vi "诊断标定4.vi"(8 "CAN端口":u16(ring), 9 "设备索引号":u16(ring), 10 "CAN卡类型":u32(ring)=4) -> ()   [LabVIEW 2013] (continued)
                                n824 = Bundle By Name(cluster=w1320, "电池串联"=w1318, "电池并联"=w1318, "电池包额定容量"=w1318, "电池包额定能量"=w1318, "电池包额定总电压"=w1318, "实际容量"=w1318, "电池厂家"=w1317, "电池类型"=w1317, "电池生产日期"=w1317) -> (w1319:T12)
                                n825 = local write "电池信息"(w1319) -> ()
                                }
                                frame "电池包组号" {
                                n826 = local read "电池信息"() -> (w1323:T12)
                                n827 = Bundle By Name(cluster=w1323, "电池包组号"="") -> (w1322:T12)
                                n828 = local write "电池信息"(w1322) -> ()
                                }
                                frame "充放电安时" {
                                w1324 = 0.0 ("累计充电总安时")
                                n829 = local read "电池信息"() -> (w1326:T12)
                                n830 = Bundle By Name(cluster=w1326, "累计充电总安时"=w1324, "累计放电总安时"=w1324) -> (w1325:T12)
                                n831 = local write "电池信息"(w1325) -> ()
                                }
                                frame "电池充放电次数" {
                                w1327 = 0.0 ("累计充电总安时")
                                n832 = local read "电池信息"() -> (w1329:T12)
                                n833 = Bundle By Name(cluster=w1329, "电池充满次数"=w1327, "电池放空次数"=w1327, "电池充电次数"=w1327) -> (w1328:T12)
                                n834 = local write "电池信息"(w1328) -> ()
                                }
                              }
                            }
                            frame "从板" {
                              n835 = case shown="\"保险位置\"" w1330 {
                                frame "假", Default {
                                }
                                frame "电压起始值" {
                                n836 = control-ref of="项目信息 2"() -> (w1331:refnum<vi>)
                                n837 = for {
                                N: 2 -> [_]
                                tunnel: [""] -> w1335 mode=indexing
                                }
                                n838 = call "表格数据输入-8.6.vi"("行数"=u32 0, "列数"=u32 1, "字符串数组"=w1335, "表格引用"=w1331) -> ()  [unwired: 8 in]
                                }
                                frame "通道电压个数" {
                                n839 = control-ref of="项目信息 2"() -> (w1337:refnum<vi>)
                                n840 = for {
                                N: 20 -> [_]
                                tunnel: [""] -> w1341 mode=indexing
                                }
                                n841 = call "表格数据输入-8.6.vi"("行数"=u32 2, "列数"=u32 1, "字符串数组"=w1341, "表格引用"=w1337) -> ()  [unwired: 8 in]
                                }
                                frame "保险位置" {
                                n842 = control-ref of="项目信息 2"() -> (w1343:refnum<vi>)
                                n843 = for {
                                N: 10 -> [_]
                                tunnel: [""] -> w1347 mode=indexing
                                }
                                n844 = call "表格数据输入-8.6.vi"("行数"=u32 24, "列数"=u32 1, "字符串数组"=w1347, "表格引用"=w1343) -> ()  [unwired: 8 in]
                                }
                                frame "温度起始值" {
                                n845 = control-ref of="项目信息 2"() -> (w1349:refnum<vi>)
                                n846 = for {
                                N: 2 -> [_]
                                tunnel: [""] -> w1353 mode=indexing
                                }
                                n847 = call "表格数据输入-8.6.vi"("行数"=u32 22, "列数"=u32 1, "字符串数组"=w1353, "表格引用"=w1349) -> ()  [unwired: 8 in]
                                }
                                frame "加热控制参数" {
                                n848 = local write "加热控制参数"(T10 {"风机开启温度"=0.0, "风机关闭温度"=0.0, "加热开启温度"=0.0, "加热关闭温度"=0.0, "风机开启温差"=0.0, "风机关闭温差"=0.0, "加热关闭温差"=0.0} ("加热控制参数")) -> ()
                                }
                                frame "一级故障阀值" {
                                n849 = local write "一级故障 6"(T14 {"电压过高"=0.0, "电压过低"=0.0, "温度过高"=0.0, "温度过低"=0.0, "电压不均衡(V)"=0.0, "温度不均衡"=0.0, "SOC过低"=0.0} ("一级故障 6")) -> ()
                                }
                                frame "二级故障阀值" {
                                n850 = local write "一级故障 7"(T14 {"电压过高"=0.0, "电压过低"=0.0, "温度过高"=0.0, "温度过低"=0.0, "电压不均衡(V)"=0.0, "温度不均衡"=0.0, "SOC过低"=0.0} ("一级故障 7")) -> ()
                                }
                                frame "三级故障阀值" {
                                n851 = local write "一级故障 8"(T14 {"电压过高"=0.0, "电压过低"=0.0, "温度过高"=0.0, "温度过低"=0.0, "电压不均衡(V)"=0.0, "温度不均衡"=0.0, "SOC过低"=0.0} ("一级故障 7")) -> ()
                                }
                              }
                            }
                          }
                        }
                        frame #1 {
                          n852 = call <vilib>:"Set Busy.vi"("disable click? (T)"=FALSE) -> ()  [unwired: 3 in, 8 out]
                          n853 = global write "EV05全局变量1.vi" "写入超时"(FALSE ("写入超时")) -> ()
                          n854 = Wait Until Next ms Multiple(millisecond multiple=u32 50 ("毫秒倍数")) -> ()  [unwired: 1 out]
                          n855 = global write "EV05全局变量1.vi" "流控帧 2"(FALSE ("流控帧 2")) -> ()
                          n856 = local write "控制1"(TRUE ("控制1")) -> ()
                          n857 = local write "写?"(FALSE ("写?")) -> ()
                          n858 = local write "消除"(TRUE ("消除")) -> ()
                        }
                        frame #2 {
                          n859 = local read "设备索引号"() -> (w1367:u16)
                          n860 = local read "CAN卡类型"() -> (w1368:u32)
                          n861 = local write "命令序号"(w1371) -> ()
                          n862 = local read "CAN端口"() -> (w1366:u16)
                          n863 = stacked-sequence {
                            tunnel: w1372 -> [_ w1383]
                            tunnel: w1371 -> [_ w1382]
                            tunnel: w1370 -> [_ w1381]
                            tunnel: w1369 -> [_ w1380]
                            tunnel: w1368 -> [w1375 w1379]
                            tunnel: w1367 -> [w1374 w1378]
                            tunnel: w1366 -> [w1373 w1377]
                            frame #0 {
                              n864 = dll-call lib="PTH1Aabs EEV05EV05监控上位机-EV05EV05data\nusbcan.dll" fn="VCI_ClearBuffer"("DeviceType"=w1375, "DeviceInd"=w1374, "CANInd"=w1373) -> (error out=w1376:errorcluster)  [unwired: 4 in, 4 out]
                              n865 = call <vilib>:"Clear Errors.vi"("error in (no error)"=w1376) -> ()  [unwired: 6 in, 1 out]
                            }
                            frame #1 {
                              n866 = call "多帧发送机制(EV05).vi"("can卡类型"=w1379, "设备索引号"=w1378, "CAN端口"=w1377, "命令"=w1383, "板号"=w1381, "命令序号"=w1382, "输入数据"=w1380) -> ()  [unwired: 1 in, 12 out]
                            }
                          }
                        }
                        frame #3 {
                          n867 = while {
                            tunnel: [w1388] -> w1385
                            tunnel: [w1387] -> w1384
                            i -> [w1391]
                            stop <- w1388 stop-if-true
                            n868 = local read "强制停止"() -> (w1386:bool)
                            n869 = global read "EV05全局变量1.vi" "写入超时"() -> (w1387:bool)
                            n870 = Greater Or Equal?(x=w1391, y=25) -> (x >= y?=w1389:bool)
                            n871 = Compound Arithmetic op=OR(w1386, w1387, w1389) -> (w1388:bool)
                            n872 = Wait Until Next ms Multiple(millisecond multiple=u32 100 ("毫秒倍数")) -> ()  [unwired: 1 out]
                          }
                        }
                        frame #4 {
                          n873 = call <vilib>:"Unset Busy.vi"() -> ()  [unwired: 2 in, 10 out]
                          n874 = case shown="假" w1394 {
                            tunnel: w1393 -> [w1395 _]
                            frame False {
                              n875 = control-ref of="结果"() -> (w1397:refnum<vi>)
                              n876 = Concatenate Strings(w1395, "     读取失败" ("字符串")) -> (w1399:string)
                              n877 = Build Array(w1399) -> (w1396:string[])
                              n878 = call "表格编辑.vi"("新元素/子数组"=w1396, "活动单元格:单元格背景色"=u32 16740749, "MCListbox引用句柄"=w1397) -> ()  [unwired: 9 out]
                            }
                            frame True {
                            }
                          }
                        }
                        frame #5 {
                          n879 = And(x=w1401, y=w1403) -> (x .and. y?=w1402:bool)
                          n880 = case shown="真" w1402 {
                            frame False {
                            }
                            frame True {
                              n881 = local write "强制停止"(FALSE ("强制停止")) -> ()
                              n882 = control-ref of="结果"() -> (w1406:refnum<vi>)
                              n883 = Concatenate Strings("读取完成" ("字符串")) -> (w1408:string)
                              n884 = Build Array(w1408) -> (w1405:string[])
                              n885 = call "表格编辑.vi"("新元素/子数组"=w1405, "活动单元格:单元格背景色"=u32 21937, "MCListbox引用句柄"=w1406) -> ()  [unwired: 9 out]
                            }
                          }
                        }
                      }
                    }
                    n886 = local read "强制停止"() -> (w1217:bool)
                    n887 = Or(x=w1217, y=w1216) -> (x .or. y?=w1214:bool)
                  }
                }
              }
              frame #2 {
                n888 = case shown="假" w1488 {
                  tunnel: w1489 -> [w1490 _]
                  frame False {
                    n889 = case shown="\"从板\"" w1490 {
                      frame "主板", Default {
                        n890 = global read "读配置文件全局.vi" "电池额定实际容量判定"() -> (w1504:bool)
                        n891 = global read "读配置文件全局.vi" "电池充放电次数判定"() -> (w1493:bool)
                        n892 = global read "读配置文件全局.vi" "加热控制参数判定"() -> (w1491:bool)
                        n893 = global read "读配置文件全局.vi" "配置文件版本判定"() -> (w1503:bool)
                        n894 = global read "读配置文件全局.vi" "充电控制参数判定"() -> (w1497:bool)
                        n895 = global read "读配置文件全局.vi" "通道电压数判定"() -> (w1509:bool)
                        n896 = global read "读配置文件全局.vi" "电压起始值判定"() -> (w1508:bool)
                        n897 = global read "读配置文件全局.vi" "温度起始值判定"() -> (w1506:bool)
                        n898 = global read "读配置文件全局.vi" "充放电安时判定"() -> (w1495:bool)
                        n899 = global read "读配置文件全局.vi" "电池包组号判定"() -> (w1494:bool)
                        n900 = global read "读配置文件全局.vi" "电池信息1判定"() -> (w1496:bool)
                        n901 = global read "读配置文件全局.vi" "从板个数判定"() -> (w1512:bool)
                        n902 = global read "读配置文件全局.vi" "产品编号判定"() -> (w1511:bool)
                        n903 = global read "读配置文件全局.vi" "电压个数判定"() -> (w1510:bool)
                        n904 = global read "读配置文件全局.vi" "温度个数判定"() -> (w1507:bool)
                        n905 = global read "读配置文件全局.vi" "保险位置判定"() -> (w1505:bool)
                        n906 = global read "读配置文件全局.vi" "一级故障判定"() -> (w1500:bool)
                        n907 = global read "读配置文件全局.vi" "二级故障判定"() -> (w1499:bool)
                        n908 = global read "读配置文件全局.vi" "三级故障判定"() -> (w1498:bool)
                        n909 = global read "读配置文件全局.vi" "车牌号判定"() -> (w1502:bool)
                        n910 = global read "读配置文件全局.vi" "SOH判定"() -> (w1501:bool)
                        n911 = Build Array(w1512, w1511, w1510, w1509, w1508, w1507, w1506, w1505, w1504, w1503, w1502, w1501, w1500, w1499, w1498, w1497, w1496, w1495, w1494, w1493, w1491) -> (w1492:bool[])
                        n912 = And Array Elements(Boolean array=w1492) -> (logical AND=w1513:bool)
                        n913 = disable-structure shown="禁用" {
                          frame Disabled {
                            n914 = global read "读配置文件全局.vi" "SOC判定"() -> ()  [unwired: 1 out]
                          }
                          frame Enabled {
                          }
                        }
                        n915 = case shown="假" w1513 {
                          tunnel: w1492 -> [_ w1518]
                          frame True {
                            n916 = control-ref of="结果"() -> (w1516:refnum<vi>)
                            n917 = Build Array("全部判定成功!!!!!!!!") -> (w1517:string[])
                            n918 = call "表格编辑.vi"("新元素/子数组"=w1517, "活动单元格:单元格背景色"=u32 6618880, "MCListbox引用句柄"=w1516) -> ()  [unwired: 9 out]
                          }
                          frame False {
                            n919 = stacked-sequence {
                              tunnel: w1518 -> [_ w1523]
                              frame #0 {
                                n920 = control-ref of="结果"() -> (w1521:refnum<vi>)
                                n921 = Build Array("全部判定失败!!!!!") -> (w1522:string[])
                                n922 = call "表格编辑.vi"("新元素/子数组"=w1522, "活动单元格:单元格背景色"=u32 16711680, "MCListbox引用句柄"=w1521) -> ()  [unwired: 9 out]
                              }
                              frame #1 {
                                n923 = for {
                                tunnel: w1523 -> [w1525] mode=indexing
                                i -> [w1524]
                                n924 = case shown="20" w1524 {
                                tunnel: w1525 -> [w1526 w1531 w1536 w1541 w1546 w1551 w1556 w1561 w1566 w1571 w1576 w1581 w1586 w1591 w1596 w1601 w1606 w1611 w1616 w1621 w1626 _]
                                frame 0 {
                                n925 = case shown="假" w1526 {
                                frame False {
                                n926 = control-ref of="结果"() -> (w1529:refnum<vi>)
                                n927 = Build Array("从板个数判定失败!") -> (w1530:string[])
                                n928 = call "表格编辑.vi"("新元素/子数组"=w1530, "活动单元格:单元格背景色"=u32 16711680, "MCListbox引用句柄"=w1529) -> ()  [unwired: 9 out]
                                }
                                frame True {
                                }
                                }
                                }
                                frame 1 {
                                n929 = case shown="假" w1531 {
                                frame False {
                                n930 = control-ref of="结果"() -> (w1534:refnum<vi>)
                                n931 = Build Array("产品编号判定失败!") -> (w1535:string[])
                                n932 = call "表格编辑.vi"("新元素/子数组"=w1535, "活动单元格:单元格背景色"=u32 16711680, "MCListbox引用句柄"=w1534) -> ()  [unwired: 9 out]
                                }
                                frame True {
                                }
                                }
                                }
                                frame 2 {
                                n933 = case shown="假" w1536 {
                                frame False {
                                n934 = control-ref of="结果"() -> (w1539:refnum<vi>)
                                n935 = Build Array("电压个数判定失败!") -> (w1540:string[])
                                n936 = call "表格编辑.vi"("新元素/子数组"=w1540, "活动单元格:单元格背景色"=u32 16711680, "MCListbox引用句柄"=w1539) -> ()  [unwired: 9 out]
                                }
                                frame True {
                                }
                                }
                                }
                                frame 3 {
                                n937 = case shown="假" w1541 {
                                frame False {
                                n938 = control-ref of="结果"() -> (w1544:refnum<vi>)
                                n939 = Build Array("通道电压数判定失败!") -> (w1545:string[])
                                n940 = call "表格编辑.vi"("新元素/子数组"=w1545, "活动单元格:单元格背景色"=u32 16711680, "MCListbox引用句柄"=w1544) -> ()  [unwired: 9 out]
                                }
                                frame True {
                                }
                                }
                                }
                                frame 4 {
                                n941 = case shown="假" w1546 {
                                frame False {
                                n942 = control-ref of="结果"() -> (w1549:refnum<vi>)
                                n943 = Build Array("电压起始值判定失败!") -> (w1550:string[])
                                n944 = call "表格编辑.vi"("新元素/子数组"=w1550, "活动单元格:单元格背景色"=u32 16711680, "MCListbox引用句柄"=w1549) -> ()  [unwired: 9 out]
                                }
                                frame True {
                                }
                                }
                                }
                                frame 5 {
                                n945 = case shown="假" w1551 {
                                frame False {
                                n946 = control-ref of="结果"() -> (w1554:refnum<vi>)
                                n947 = Build Array("温度个数判定失败!") -> (w1555:string[])
                                n948 = call "表格编辑.vi"("新元素/子数组"=w1555, "活动单元格:单元格背景色"=u32 16711680, "MCListbox引用句柄"=w1554) -> ()  [unwired: 9 out]
                                }
                                frame True {
                                }
                                }
                                }
                                frame 6 {
                                n949 = case shown="假" w1556 {
                                frame False {
                                n950 = control-ref of="结果"() -> (w1559:refnum<vi>)
                                n951 = Build Array("温度起始值判定失败!") -> (w1560:string[])
                                n952 = call "表格编辑.vi"("新元素/子数组"=w1560, "活动单元格:单元格背景色"=u32 16711680, "MCListbox引用句柄"=w1559) -> ()  [unwired: 9 out]
                                }
                                frame True {
                                }
                                }
                                }
                                frame 7 {
                                n953 = case shown="假" w1561 {
                                frame False {
                                n954 = control-ref of="结果"() -> (w1564:refnum<vi>)
                                n955 = Build Array("保险位置判定失败!") -> (w1565:string[])
                                n956 = call "表格编辑.vi"("新元素/子数组"=w1565, "活动单元格:单元格背景色"=u32 16711680, "MCListbox引用句柄"=w1564) -> ()  [unwired: 9 out]
                                }
                                frame True {
                                }
                                }
                                }
                                frame 8 {
                                n957 = case shown="假" w1566 {
                                frame False {
                                n958 = control-ref of="结果"() -> (w1569:refnum<vi>)
                                n959 = Build Array("电池额定实际容量判定失败!") -> (w1570:string[])
                                n960 = call "表格编辑.vi"("新元素/子数组"=w1570, "活动单元格:单元格背景色"=u32 16711680, "MCListbox引用句柄"=w1569) -> ()  [unwired: 9 out]
                                }
                                frame True {
                                }
                                }
                                }
                                frame 9 {
                                n961 = case shown="假" w1571 {
                                frame False {
                                n962 = control-ref of="结果"() -> (w1574:refnum<vi>)
                                n963 = Build Array("配置文件版本判定失败!") -> (w1575:string[])
                                n964 = call "表格编辑.vi"("新元素/子数组"=w1575, "活动单元格:单元格背景色"=u32 16711680, "MCListbox引用句柄"=w1574) -> ()  [unwired: 9 out]
                                }
                                frame True {
                                }
                                }
                                }
                                frame 10 {
                                n965 = case shown="假" w1576 {
                                frame False {
                                n966 = control-ref of="结果"() -> (w1579:refnum<vi>)
                                n967 = Build Array("车牌号判定失败!") -> (w1580:string[])
                                n968 = call "表格编辑.vi"("新元素/子数组"=w1580, "活动单元格:单元格背景色"=u32 16711680, "MCListbox引用句柄"=w1579) -> ()  [unwired: 9 out]
                                }
                                frame True {
                                }
                                }
                                }
                                frame 11 {
                                n969 = case shown="假" w1581 {
                                frame False {
                                n970 = control-ref of="结果"() -> (w1584:refnum<vi>)
                                n971 = Build Array("SOH判定失败!") -> (w1585:string[])
                                n972 = call "表格编辑.vi"("新元素/子数组"=w1585, "活动单元格:单元格背景色"=u32 16711680, "MCListbox引用句柄"=w1584) -> ()  [unwired: 9 out]
                                }
                                frame True {
                                }
                                }
                                }
                                frame 12 {
                                n973 = case shown="假" w1586 {
                                frame False {
                                n974 = control-ref of="结果"() -> (w1589:refnum<vi>)
                                n975 = Build Array("一级故障阀值判定失败!") -> (w1590:string[])
                                n976 = call "表格编辑.vi"("新元素/子数组"=w1590, "活动单元格:单元格背景色"=u32 16711680, "MCListbox引用句柄"=w1589) -> ()  [unwired: 9 out]
                                }
                                frame True {
                                }
                                }
                                }
                                frame 13 {
                                n977 = case shown="假" w1591 {
                                frame False {
                                n978 = control-ref of="结果"() -> (w1594:refnum<vi>)
                                n979 = Build Array("二级故障阀值判定失败!") -> (w1595:string[])
                                n980 = call "表格编辑.vi"("新元素/子数组"=w1595, "活动单元格:单元格背景色"=u32 16711680, "MCListbox引用句柄"=w1594) -> ()  [unwired: 9 out]
                                }
                                frame True {
                                }
                                }
                                }
                                frame 14 {
                                n981 = case shown="假" w1596 {
                                frame False {
                                n982 = control-ref of="结果"() -> (w1599:refnum<vi>)
                                n983 = Build Array("三级故障阀值判定失败!") -> (w1600:string[])
                                n984 = call "表格编辑.vi"("新元素/子数组"=w1600, "活动单元格:单元格背景色"=u32 16711680, "MCListbox引用句柄"=w1599) -> ()  [unwired: 9 out]
                                }
                                frame True {
                                }
                                }
                                }
                                frame 15 {
                                n985 = case shown="假" w1601 {
                                frame False {
                                n986 = control-ref of="结果"() -> (w1604:refnum<vi>)
                                n987 = Build Array("充电控制参数判定失败!") -> (w1605:string[])
                                n988 = call "表格编辑.vi"("新元素/子数组"=w1605, "活动单元格:单元格背景色"=u32 16711680, "MCListbox引用句柄"=w1604) -> ()  [unwired: 9 out]
                                }
                                frame True {
                                }
                                }
                                }
                                frame 16 {
                                n989 = case shown="假" w1606 {
                                frame False {
                                n990 = control-ref of="结果"() -> (w1609:refnum<vi>)
                                n991 = Build Array("电池信息1判定失败!") -> (w1610:string[])
                                n992 = call "表格编辑.vi"("新元素/子数组"=w1610, "活动单元格:单元格背景色"=u32 16711680, "MCListbox引用句柄"=w1609) -> ()  [unwired: 9 out]
                                }
                                frame True {
                                }
                                }
                                }
                                frame 17 {
                                n993 = case shown="假" w1611 {
                                frame False {
                                n994 = control-ref of="结果"() -> (w1614:refnum<vi>)
                                n995 = Build Array("充放电安时判定失败!") -> (w1615:string[])
                                n996 = call "表格编辑.vi"("新元素/子数组"=w1615, "活动单元格:单元格背景色"=u32 16711680, "MCListbox引用句柄"=w1614) -> ()  [unwired: 9 out]
                                }
                                frame True {
                                }
                                }
                                }
                                frame 18 {
                                n997 = case shown="假" w1616 {
                                frame False {
                                n998 = control-ref of="结果"() -> (w1619:refnum<vi>)
                                n999 = Build Array("电池包组号判定失败!") -> (w1620:string[])
                                n1000 = call "表格编辑.vi"("新元素/子数组"=w1620, "活动单元格:单元格背景色"=u32 16711680, "MCListbox引用句柄"=w1619) -> ()  [unwired: 9 out]
                                }
                                frame True {
                                }
                                }
                                }
                                frame 19 {
                                n1001 = case shown="假" w1621 {
                                frame False {
                                n1002 = control-ref of="结果"() -> (w1624:refnum<vi>)
                                n1003 = Build Array("电池充放电次数判定失败!") -> (w1625:string[])
                                n1004 = call "表格编辑.vi"("新元素/子数组"=w1625, "活动单元格:单元格背景色"=u32 16711680, "MCListbox引用句柄"=w1624) -> ()  [unwired: 9 out]
                                }
                                frame True {
                                }
                                }
                                }
                                frame 20 {
                                n1005 = case shown="假" w1626 {
                                frame False {
                                n1006 = control-ref of="结果"() -> (w1629:refnum<vi>)
                                n1007 = Build Array("加热控制参数判定失败!") -> (w1630:string[])
                                n1008 = call "表格编辑.vi"("新元素/子数组"=w1630, "活动单元格:单元格背景色"=u32 16711680, "MCListbox引用句柄"=w1629) -> ()  [unwired: 9 out]
                                }
                                frame True {
                                }
                                }
                                }
                                frame 99, Default {
                                }
                                }
                                }
                              }
                            }
                          }
                        }
                      }
                      frame "从板" {
                        n1009 = global read "读配置文件全局2.vi" "电压起始值判定"() -> (w1639:bool)
                        n1010 = global read "读配置文件全局2.vi" "温度起始值判定"() -> (w1636:bool)
                        n1011 = global read "读配置文件全局2.vi" "加热控制参数判定"() -> (w1631:bool)
                        n1012 = global read "读配置文件全局2.vi" "通道电压判定"() -> (w1638:bool)
                        n1013 = global read "读配置文件全局2.vi" "保险位置判定"() -> (w1637:bool)
                        n1014 = global read "读配置文件全局2.vi" "一级故障判定"() -> (w1634:bool)
                        n1015 = global read "读配置文件全局2.vi" "二级故障判定"() -> (w1633:bool)
                        n1016 = global read "读配置文件全局2.vi" "三级故障判定"() -> (w1632:bool)
                        n1017 = global read "读配置文件全局2.vi" "从板号判定"() -> (w1640:bool)
                        n1018 = Build Array(w1640, w1639, w1638, w1637, w1636, w1634, w1633, w1632, w1631) -> (w1635:bool[])
                        n1019 = And Array Elements(Boolean array=w1635) -> (logical AND=w1641:bool)
                        n1020 = case shown="假" w1641 {
                          tunnel: w1635 -> [_ w1646]
                          frame True {
                            n1021 = control-ref of="结果"() -> (w1644:refnum<vi>)
                            n1022 = Build Array("读取判定成功!!!!!!!!") -> (w1645:string[])
                            n1023 = call "表格编辑.vi"("新元素/子数组"=w1645, "活动单元格:单元格背景色"=u32 6618880, "MCListbox引用句柄"=w1644) -> ()  [unwired: 9 out]
                          }
                          frame False {
                            n1024 = stacked-sequence {
                              tunnel: w1646 -> [_ w1651]
                              frame #0 {
                                n1025 = control-ref of="结果"() -> (w1649:refnum<vi>)
                                n1026 = Build Array("读取判定失败!!!!!") -> (w1650:string[])
                                n1027 = call "表格编辑.vi"("新元素/子数组"=w1650, "活动单元格:单元格背景色"=u32 16711680, "MCListbox引用句柄"=w1649) -> ()  [unwired: 9 out]
                              }
                              frame #1 {
                                n1028 = for {
                                tunnel: w1651 -> [w1652] mode=indexing
                                i -> [w1653]
                                n1029 = case shown="0" w1653 {
                                tunnel: w1652 -> [w1654 w1659 w1664 w1669 w1674 w1679 w1684 w1689 w1694 _]
                                frame 0 {
                                n1030 = case shown="假" w1654 {
                                frame False {
                                n1031 = control-ref of="结果"() -> (w1657:refnum<vi>)
                                n1032 = Build Array("从板号判定失败!") -> (w1658:string[])
                                n1033 = call "表格编辑.vi"("新元素/子数组"=w1658, "活动单元格:单元格背景色"=u32 16711680, "MCListbox引用句柄"=w1657) -> ()  [unwired: 9 out]
                                }
                                frame True {
                                }
                                }
                                }
                                frame 1 {
                                n1034 = case shown="假" w1659 {
                                frame False {
                                n1035 = control-ref of="结果"() -> (w1662:refnum<vi>)
                                n1036 = Build Array("电压起始值判定失败!") -> (w1663:string[])
                                n1037 = call "表格编辑.vi"("新元素/子数组"=w1663, "活动单元格:单元格背景色"=u32 16711680, "MCListbox引用句柄"=w1662) -> ()  [unwired: 9 out]
                                }
                                frame True {
                                }
                                }
                                }
                                frame 2 {
                                n1038 = case shown="假" w1664 {
                                frame False {
                                n1039 = control-ref of="结果"() -> (w1667:refnum<vi>)
                                n1040 = Build Array("通道电压节数判定失败!") -> (w1668:string[])
                                n1041 = call "表格编辑.vi"("新元素/子数组"=w1668, "活动单元格:单元格背景色"=u32 16711680, "MCListbox引用句柄"=w1667) -> ()  [unwired: 9 out]
                                }
                                frame True {
                                }
                                }
                                }
                                frame 3 {
                                n1042 = case shown="假" w1669 {
                                frame False {
                                n1043 = control-ref of="结果"() -> (w1672:refnum<vi>)
                                n1044 = Build Array("保险位置判定失败!") -> (w1673:string[])
                                n1045 = call "表格编辑.vi"("新元素/子数组"=w1673, "活动单元格:单元格背景色"=u32 16711680, "MCListbox引用句柄"=w1672) -> ()  [unwired: 9 out]
                                }
                                frame True {
                                }
                                }
                                }
                                frame 4 {
                                n1046 = case shown="假" w1674 {
                                frame False {
                                n1047 = control-ref of="结果"() -> (w1677:refnum<vi>)
                                n1048 = Build Array("温度起始值判定失败!") -> (w1678:string[])
                                n1049 = call "表格编辑.vi"("新元素/子数组"=w1678, "活动单元格:单元格背景色"=u32 16711680, "MCListbox引用句柄"=w1677) -> ()  [unwired: 9 out]
                                }
                                frame True {
                                }
                                }
                                }
                                frame 5 {
                                n1050 = case shown="假" w1679 {
                                frame False {
                                n1051 = control-ref of="结果"() -> (w1682:refnum<vi>)
                                n1052 = Build Array("一级故障判定失败!") -> (w1683:string[])
                                n1053 = call "表格编辑.vi"("新元素/子数组"=w1683, "活动单元格:单元格背景色"=u32 16711680, "MCListbox引用句柄"=w1682) -> ()  [unwired: 9 out]
                                }
                                frame True {
                                }
                                }
                                }
                                frame 6 {
                                n1054 = case shown="假" w1684 {
                                frame False {
                                n1055 = control-ref of="结果"() -> (w1687:refnum<vi>)
                                n1056 = Build Array("二级故障判定失败!") -> (w1688:string[])
                                n1057 = call "表格编辑.vi"("新元素/子数组"=w1688, "活动单元格:单元格背景色"=u32 16711680, "MCListbox引用句柄"=w1687) -> ()  [unwired: 9 out]
                                }
                                frame True {
                                }
                                }
                                }
                                frame 7 {
                                n1058 = case shown="假" w1689 {
                                frame False {
                                n1059 = control-ref of="结果"() -> (w1692:refnum<vi>)
                                n1060 = Build Array("三级故障判定失败!") -> (w1693:string[])
                                n1061 = call "表格编辑.vi"("新元素/子数组"=w1693, "活动单元格:单元格背景色"=u32 16711680, "MCListbox引用句柄"=w1692) -> ()  [unwired: 9 out]
                                }
                                frame True {
                                }
                                }
                                }
                                frame 8 {
                                n1062 = case shown="假" w1694 {
                                frame False {
                                n1063 = control-ref of="结果"() -> (w1697:refnum<vi>)
                                n1064 = Build Array("加热控制参数判定失败!") -> (w1698:string[])
                                n1065 = call "表格编辑.vi"("新元素/子数组"=w1698, "活动单元格:单元格背景色"=u32 16711680, "MCListbox引用句柄"=w1697) -> ()  [unwired: 9 out]
                                }
                                frame True {
                                }
                                }
                                }
                                frame 99, Default {
                                }
                                }
                                }
                              }
                            }
                          }
                        }
                        n1066 = disable-structure shown="禁用" {
                          frame Disabled {
                            n1067 = global read "读配置文件全局.vi" "SOC判定"() -> ()  [unwired: 1 out]
                          }
                          frame Enabled {
                          }
                        }
                      }
                    }
                  }
                  frame True {
                  }
                }
              }
            }
            n1068 = stacked-sequence {
              tunnel: w1000 -> [_]
              frame #0 {
                n1069 = local write "强制停止"(FALSE ("强制停止")) -> ()
              }
            }
          }
          frame "开启均衡" {
            n1070 = local read "从板板号"() -> (w1699:u8)
            n1071 = stacked-sequence {
              tunnel: 133 -> [_ w1720 _ _]
              tunnel: w1699 -> [_ _ _ _]
              frame #0 {
                w1708 = u8 0 items=["Normal", "Listen Only"] ("工作方式")
                w1707 = u8 1 items=["Dual Filter", "Single Filter"] ("滤波方式")
                n1072 = global write "EV05全局变量1.vi" "读取超时"(FALSE ("读取超时")) -> ()
                n1073 = global write "EV05全局变量1.vi" "流控帧 2"(FALSE ("流控帧 2")) -> ()
                n1074 = local write "写?"(TRUE ("写?")) -> ()
                n1075 = local read "设备索引号"() -> (w1703:u16)
                n1076 = local read "CAN卡类型"() -> (w1702:u32)
                n1077 = local read "CAN端口"() -> (w1704:u16)
                n1078 = local write "控制1"(TRUE ("控制1")) -> ()
                n1079 = local write "消除"(TRUE ("消除")) -> ()
                n1080 = call "CAN_Init-8.6.vi"("CAN卡类型"=w1702, "设备索引号"=w1703, "CAN端口"=w1704, "操作类型"=enum16{"初始化CAN", "关闭CAN"}."初始化CAN", "滤波方式"=w1707, "Accept Code"=u32 606601216, "簇"=T20 {"打开CAN"=FALSE, "初始化CAN"=TRUE, "开始CAN"=TRUE, "重启"=FALSE, "关闭CAN"=FALSE}, "Mask Code"=u32 524287 ("Accept Code"), "工作方式"=w1708, "是否滤波"=TRUE, "滤波选择"=T19 {"fiter_mode"=1, "fiter_endid"=75825152, "fiter_startid"=75890687}) -> ()  [unwired: 3 in, 6 out]
                n1081 = Wait Until Next ms Multiple(millisecond multiple=u32 20 ("毫秒倍数")) -> ()  [unwired: 1 out]
              }
              frame #1 {
                n1082 = local write "命令"(w1720) -> ()
                n1083 = call "ID组合.vi"("SA(4)"=0 ("PDU(1)"), "PS(3)"=63 ("PDU(1)"), "PF(2)"=w1720, "PDU(1)"=4) -> ("ID"=w1719:i32)  [unwired: 7 out]
                n1084 = local read "从板板号"() -> (w1731:u8)
                n1085 = local write "命令序号"(2) -> ()
                n1086 = local read "设备索引号"() -> (w1725:u16)
                n1087 = local read "CAN卡类型"() -> (w1726:u32)
                n1088 = local read "CAN端口"() -> (w1724:u16)
                n1089 = Add(x=w1731, y=1) -> (x+y=w1729:i32)
                n1090 = Build Array(2, 2, w1729) -> (w1727:i32[])
                n1091 = call "transmit-8.6.vi"("can卡类型"=w1726, "设备索引号"=w1725, "CAN端口"=w1724, "ID"=w1719, "Data"=w1727) -> ()  [unwired: 2 in, 13 out]
              }
              frame #2 {
                n1092 = Wait Until Next ms Multiple(millisecond multiple=u32 1000 ("毫秒倍数")) -> ()  [unwired: 1 out]
              }
              frame #3 {
                w1738 = u8 0 items=["Normal", "Listen Only"] ("工作方式")
                w1739 = u8 1 items=["Dual Filter", "Single Filter"] ("滤波方式")
                n1093 = global write "EV05全局变量1.vi" "流控帧 2"(FALSE ("流控帧 2")) -> ()
                n1094 = local read "设备索引号"() -> (w1743:u16)
                n1095 = local read "CAN卡类型"() -> (w1744:u32)
                n1096 = local write "控制1"(FALSE ("控制1")) -> ()
                n1097 = local read "CAN端口"() -> (w1742:u16)
                n1098 = local write "消除"(FALSE ("消除")) -> ()
                n1099 = call <vilib>:"Unset Busy.vi"() -> ()  [unwired: 2 in, 10 out]
                n1100 = call "CAN_Init-8.6.vi"("CAN卡类型"=w1744, "设备索引号"=w1743, "CAN端口"=w1742, "操作类型"=enum16{"初始化CAN", "关闭CAN"}."初始化CAN", "滤波方式"=w1739, "Accept Code"=u32 3221225472, "簇"=T20 {"打开CAN"=FALSE, "初始化CAN"=TRUE, "开始CAN"=TRUE, "重启"=FALSE, "关闭CAN"=FALSE}, "Mask Code"=u32 1073741823 ("Accept Code"), "工作方式"=w1738, "是否滤波"=TRUE, "滤波选择"=T19 {"fiter_mode"=1, "fiter_endid"=402653184, "fiter_startid"=419430399}) -> ()  [unwired: 3 in, 6 out]
              }
            }
          }
          frame "关闭均衡" {
            n1101 = local read "从板板号"() -> (w1748:u8)
            n1102 = stacked-sequence {
              tunnel: 133 -> [_ w1770 _ _]
              tunnel: w1748 -> [_ _ _ _]
              frame #0 {
                w1757 = u8 0 items=["Normal", "Listen Only"] ("工作方式")
                w1756 = u8 1 items=["Dual Filter", "Single Filter"] ("滤波方式")
                n1103 = global write "EV05全局变量1.vi" "读取超时"(FALSE ("读取超时")) -> ()
                n1104 = global write "EV05全局变量1.vi" "流控帧 2"(FALSE ("流控帧 2")) -> ()
                n1105 = local write "写?"(TRUE ("写?")) -> ()
                n1106 = local read "设备索引号"() -> (w1752:u16)
                n1107 = local read "CAN卡类型"() -> (w1751:u32)
                n1108 = local read "CAN端口"() -> (w1753:u16)
                n1109 = local write "控制1"(TRUE ("控制1")) -> ()
                n1110 = local write "消除"(TRUE ("消除")) -> ()
                n1111 = call "CAN_Init-8.6.vi"("CAN卡类型"=w1751, "设备索引号"=w1752, "CAN端口"=w1753, "操作类型"=enum16{"初始化CAN", "关闭CAN"}."初始化CAN", "滤波方式"=w1756, "Accept Code"=u32 606601216, "簇"=T20 {"打开CAN"=FALSE, "初始化CAN"=TRUE, "开始CAN"=TRUE, "重启"=FALSE, "关闭CAN"=FALSE}, "Mask Code"=u32 524287 ("Accept Code"), "工作方式"=w1757, "是否滤波"=TRUE, "滤波选择"=T19 {"fiter_mode"=1, "fiter_endid"=75825152, "fiter_startid"=75890687}) -> ()  [unwired: 3 in, 6 out]
                n1112 = Wait Until Next ms Multiple(millisecond multiple=u32 20 ("毫秒倍数")) -> ()  [unwired: 1 out]
              }
              frame #1 {
                n1113 = local write "命令"(w1770) -> ()
                n1114 = call "ID组合.vi"("SA(4)"=0 ("PDU(1)"), "PS(3)"=63 ("PDU(1)"), "PF(2)"=w1770, "PDU(1)"=4) -> ("ID"=w1769:i32)  [unwired: 7 out]
                n1115 = local read "均衡类型选择"() -> (w1780:enum16{"放电均衡", "充电均衡", "充放电均衡"})
                n1116 = local write "命令序号"(3) -> ()
                n1117 = local read "设备索引号"() -> (w1775:u16)
                n1118 = local read "CAN卡类型"() -> (w1776:u32)
                n1119 = local read "CAN端口"() -> (w1774:u16)
                n1120 = Add(x=w1780, y=1) -> (x+y=w1778:i32)
                n1121 = Build Array(2, 3, w1778) -> (w1777:i32[])
                n1122 = call "transmit-8.6.vi"("can卡类型"=w1776, "设备索引号"=w1775, "CAN端口"=w1774, "ID"=w1769, "Data"=w1777) -> ()  [unwired: 2 in, 13 out]
              }
              frame #2 {
                n1123 = Wait Until Next ms Multiple(millisecond multiple=u32 1000 ("毫秒倍数")) -> ()  [unwired: 1 out]
              }
              frame #3 {
                w1787 = u8 0 items=["Normal", "Listen Only"] ("工作方式")
                w1788 = u8 1 items=["Dual Filter", "Single Filter"] ("滤波方式")
                n1124 = local read "设备索引号"() -> (w1792:u16)
                n1125 = local read "CAN卡类型"() -> (w1793:u32)
                n1126 = global write "EV05全局变量1.vi" "流控帧 2"(FALSE ("流控帧 2")) -> ()
                n1127 = local read "CAN端口"() -> (w1791:u16)
                n1128 = local write "控制1"(FALSE ("控制1")) -> ()
                n1129 = local write "消除"(FALSE ("消除")) -> ()
                n1130 = call "CAN_Init-8.6.vi"("CAN卡类型"=w1793, "设备索引号"=w1792, "CAN端口"=w1791, "操作类型"=enum16{"初始化CAN", "关闭CAN"}."初始化CAN", "滤波方式"=w1788, "Accept Code"=u32 3221225472, "簇"=T20 {"打开CAN"=FALSE, "初始化CAN"=TRUE, "开始CAN"=TRUE, "重启"=FALSE, "关闭CAN"=FALSE}, "Mask Code"=u32 1073741823 ("Accept Code"), "工作方式"=w1787, "是否滤波"=TRUE, "滤波选择"=T19 {"fiter_mode"=1, "fiter_endid"=402653184, "fiter_startid"=419430399}) -> ()  [unwired: 3 in, 6 out]
                n1131 = call <vilib>:"Unset Busy.vi"() -> ()  [unwired: 2 in, 10 out]
              }
            }
          }
          frame "强制均衡" {
            n1132 = local read "从板板号"() -> (w1797:u8)
            n1133 = stacked-sequence {
              tunnel: 133 -> [_ w1819 _ _]
              tunnel: w1797 -> [_ _ _ _]
              frame #0 {
                w1806 = u8 0 items=["Normal", "Listen Only"] ("工作方式")
                w1805 = u8 1 items=["Dual Filter", "Single Filter"] ("滤波方式")
                n1134 = global write "EV05全局变量1.vi" "读取超时"(FALSE ("读取超时")) -> ()
                n1135 = global write "EV05全局变量1.vi" "流控帧 2"(FALSE ("流控帧 2")) -> ()
                n1136 = local write "写?"(TRUE ("写?")) -> ()
                n1137 = local read "设备索引号"() -> (w1801:u16)
                n1138 = local read "CAN卡类型"() -> (w1800:u32)
                n1139 = local write "控制1"(TRUE ("控制1")) -> ()
                n1140 = local read "CAN端口"() -> (w1802:u16)
                n1141 = local write "消除"(TRUE ("消除")) -> ()
                n1142 = call "CAN_Init-8.6.vi"("CAN卡类型"=w1800, "设备索引号"=w1801, "CAN端口"=w1802, "操作类型"=enum16{"初始化CAN", "关闭CAN"}."初始化CAN", "滤波方式"=w1805, "Accept Code"=u32 606601216, "簇"=T20 {"打开CAN"=FALSE, "初始化CAN"=TRUE, "开始CAN"=TRUE, "重启"=FALSE, "关闭CAN"=FALSE}, "Mask Code"=u32 524287 ("Accept Code"), "工作方式"=w1806, "是否滤波"=TRUE, "滤波选择"=T19 {"fiter_mode"=1, "fiter_endid"=75825152, "fiter_startid"=75890687}) -> ()  [unwired: 3 in, 6 out]
                n1143 = Wait Until Next ms Multiple(millisecond multiple=u32 20 ("毫秒倍数")) -> ()  [unwired: 1 out]
              }
              frame #1 {
                n1144 = local read "强制类型"() -> (w1827:enum16{"全通道开启", "清待均衡时间"})
                n1145 = local write "命令"(w1819) -> ()
                n1146 = call "ID组合.vi"("SA(4)"=0 ("PDU(1)"), "PS(3)"=63 ("PDU(1)"), "PF(2)"=w1819, "PDU(1)"=4) -> ("ID"=w1818:i32)  [unwired: 7 out]
                n1147 = case shown="\"全通道开启\", 默认" w1827 {
                  tunnel: [4 254] -> w1826
                  frame "全通道开启", Default {
                  }
                  frame "清待均衡时间" {
                  }
                }
                n1148 = local read "设备索引号"() -> (w1823:u16)
                n1149 = local read "CAN卡类型"() -> (w1824:u32)
                n1150 = local write "命令序号"(4) -> ()
                n1151 = local read "CAN端口"() -> (w1822:u16)
                n1152 = Build Array(2, w1826, 1) -> (w1825:i32[])
                n1153 = call "transmit-8.6.vi"("can卡类型"=w1824, "设备索引号"=w1823, "CAN端口"=w1822, "ID"=w1818, "Data"=w1825) -> ()  [unwired: 2 in, 13 out]
              }
              frame #2 {
                n1154 = Wait Until Next ms Multiple(millisecond multiple=u32 1000 ("毫秒倍数")) -> ()  [unwired: 1 out]
              }
              frame #3 {
                w1840 = u8 0 items=["Normal", "Listen Only"] ("工作方式")
                w1839 = u8 1 items=["Dual Filter", "Single Filter"] ("滤波方式")
                n1155 = global write "EV05全局变量1.vi" "流控帧 2"(FALSE ("流控帧 2")) -> ()
                n1156 = local write "控制1"(FALSE ("控制1")) -> ()
                n1157 = local read "设备索引号"() -> (w1835:u16)
                n1158 = local read "CAN卡类型"() -> (w1834:u32)
                n1159 = local write "消除"(FALSE ("消除")) -> ()
                n1160 = local read "CAN端口"() -> (w1836:u16)
                n1161 = call <vilib>:"Unset Busy.vi"() -> ()  [unwired: 2 in, 10 out]
                n1162 = call "CAN_Init-8.6.vi"("CAN卡类型"=w1834, "设备索引号"=w1835, "CAN端口"=w1836, "操作类型"=enum16{"初始化CAN", "关闭CAN"}."初始化CAN", "滤波方式"=w1839, "Accept Code"=u32 3221225472, "簇"=T20 {"打开CAN"=FALSE, "初始化CAN"=TRUE, "开始CAN"=TRUE, "重启"=FALSE, "关闭CAN"=FALSE}, "Mask Code"=u32 1073741823 ("Accept Code"), "工作方式"=w1840, "是否滤波"=TRUE, "滤波选择"=T19 {"fiter_mode"=1, "fiter_endid"=402653184, "fiter_startid"=419430399}) -> ()  [unwired: 3 in, 6 out]
              }
            }
          }
          frame "项目软件版本读取" {
            n1163 = stacked-sequence {
              seq-local: [_ w1861 _] -> [_ _ w1868]
              frame #0 {
                n1164 = local read "设备索引号"() -> (w1848:u16)
                n1165 = local read "CAN卡类型"() -> (w1849:u32)
                n1166 = local read "CAN端口"() -> (w1847:u16)
                n1167 = stacked-sequence {
                  tunnel: w1849 -> [w1852 w1860]
                  tunnel: w1848 -> [w1851 w1859]
                  tunnel: w1847 -> [w1850 w1858]
                  frame #0 {
                    n1168 = dll-call lib="PTH1Aabs EEV05EV05监控上位机-EV05EV05data\nusbcan.dll" fn="VCI_ClearBuffer"("DeviceType"=w1852, "DeviceInd"=w1851, "CANInd"=w1850) -> (error out=w1853:errorcluster)  [unwired: 4 in, 4 out]
                    n1169 = call <vilib>:"Clear Errors.vi"("error in (no error)"=w1853) -> ()  [unwired: 6 in, 1 out]
                  }
                  frame #1 {
                    w1857 = u8 137 ("命令")
                    w1856 = u32 1 ("命令序号")
                    n1170 = local read "从板板号"() -> (w1854:u8)
                    n1171 = local write "命令"(w1857) -> ()
                    n1172 = call "多帧发送机制(EV05).vi"("can卡类型"=w1860, "设备索引号"=w1859, "CAN端口"=w1858, "命令"=w1857, "板号"=w1854, "命令序号"=w1856, "输入数据"=dbl[] [0.0]) -> ()  [unwired: 1 in, 12 out]
                    n1173 = local write "命令序号"(w1856) -> ()
                  }
                }
              }
              frame #1 {
                n1174 = while {
                  tunnel: [w1862] -> w1861
                  i -> [w1867]
                  stop <- w1864 stop-if-true
                  n1175 = global read "EV05全局变量1.vi" "写入超时"() -> (w1862:bool)
                  n1176 = Greater Or Equal?(x=w1867, y=25) -> (x >= y?=w1865:bool)
                  n1177 = Or(x=w1862, y=w1865) -> (x .or. y?=w1864:bool)
                  n1178 = Wait Until Next ms Multiple(millisecond multiple=u32 100 ("毫秒倍数")) -> ()  [unwired: 1 out]
                }
              }
              frame #2 {
                n1179 = case shown="假" w1868 {
                  frame False {
                    n1180 = control-ref of="结果"() -> (w1870:refnum<vi>)
                    n1181 = Concatenate Strings("项目软件版本" ("字符串"), "     读取失败" ("字符串")) -> (w1873:string)
                    n1182 = Build Array(w1873) -> (w1872:string[])
                    n1183 = call "表格编辑(版本读取).vi"("新元素/子数组"=w1872, "活动单元格:单元格背景色"=u32 16740749, "MCListbox引用句柄"=w1870) -> ()  [unwired: 9 out]
                  }
                  frame True {
                  }
                }
                n1184 = call <vilib>:"Unset Busy.vi"() -> ()  [unwired: 2 in, 10 out]
              }
            }
          }
          frame "读取故障状态" {
            n1185 = stacked-sequence {
              seq-local: [_ w1897 _] -> [_ _ w1904]
              frame #0 {
                n1186 = local read "设备索引号"() -> (w1876:u16)
                n1187 = local read "CAN卡类型"() -> (w1877:u32)
                n1188 = local read "CAN端口"() -> (w1875:u16)
                n1189 = stacked-sequence {
                  tunnel: w1877 -> [w1880 w1889]
                  tunnel: w1876 -> [w1879 w1888]
                  tunnel: w1875 -> [w1878 w1887]
                  frame #0 {
                    n1190 = dll-call lib="PTH1Aabs EEV05EV05监控上位机-EV05EV05data\nusbcan.dll" fn="VCI_ClearBuffer"("DeviceType"=w1880, "DeviceInd"=w1879, "CANInd"=w1878) -> (error out=w1881:errorcluster)  [unwired: 4 in, 4 out]
                    n1191 = call <vilib>:"Clear Errors.vi"("error in (no error)"=w1881) -> ()  [unwired: 6 in, 1 out]
                  }
                  frame #1 {
                    w1886 = u8 133 ("命令")
                    n1192 = local read "状态选择"() -> (w1883:T18)
                    n1193 = local read "从板板号 2"() -> (w1884:u8)
                    n1194 = local write "命令"(w1886) -> ()
                    n1195 = case shown="\"预充电故障,继电器驱动故障\"" w1883 {
                      tunnel: [1 2 3 4 5 6 7] -> w1882
                      frame "电压,内总电压,外总电压,温度,电流,绝缘,系统时钟,充电均衡,放电均衡", Default {
                      }
                      frame "CPU,CPU内部EE存储器,CPU内部FLASH,内部EE存储器,45db存储器" {
                      }
                      frame "CAN检测故障" {
                      }
                      frame "软件故障" {
                      }
                      frame "RS485,RS232检测故障" {
                      }
                      frame "DI,DO,AI,AO检测故障" {
                      }
                      frame "预充电故障,继电器驱动故障" {
                      }
                    }
                    n1196 = call "多帧发送机制(EV05).vi"("can卡类型"=w1889, "设备索引号"=w1888, "CAN端口"=w1887, "命令"=w1886, "板号"=w1884, "命令序号"=w1882, "输入数据"=dbl[] [0.0]) -> ()  [unwired: 1 in, 12 out]
                    n1197 = local write "命令序号"(w1882) -> ()
                  }
                }
              }
              frame #1 {
                n1198 = while {
                  tunnel: [w1898] -> w1897
                  i -> [w1903]
                  stop <- w1900 stop-if-true
                  n1199 = global read "EV05全局变量1.vi" "写入超时"() -> (w1898:bool)
                  n1200 = Greater Or Equal?(x=w1903, y=25) -> (x >= y?=w1901:bool)
                  n1201 = Or(x=w1898, y=w1901) -> (x .or. y?=w1900:bool)
                  n1202 = Wait Until Next ms Multiple(millisecond multiple=u32 100 ("毫秒倍数")) -> ()  [unwired: 1 out]
                }
              }
              frame #2 {
                n1203 = case shown="真" w1904 {
                  frame False {
                    n1204 = Concatenate Strings("故障信息" ("字符串"), "     读取失败" ("字符串")) -> (w1906:string)
                    n1205 = One Button Dialog(message=w1906, button name ("OK")="确定" ("按钮名称（“确定”）")) -> ()  [unwired: 1 out]
                  }
                  frame True {
                    n1206 = One Button Dialog(message="故障信息读取完成" ("字符串"), button name ("OK")="确定" ("按钮名称（“确定”）")) -> ()  [unwired: 1 out]
                  }
                }
                n1207 = call <vilib>:"Unset Busy.vi"() -> ()  [unwired: 2 in, 10 out]
              }
            }
          }
          frame "平台软件版本读取" {
            n1208 = stacked-sequence {
              seq-local: [_ w1926 _] -> [_ _ w1933]
              frame #0 {
                n1209 = local read "设备索引号"() -> (w1913:u16)
                n1210 = local read "CAN卡类型"() -> (w1914:u32)
                n1211 = local read "CAN端口"() -> (w1912:u16)
                n1212 = stacked-sequence {
